vi "TimeLmtDialog.vi"(9 "time(s)":i32=5, 10 "Infoin":string="在这里填写显示的信息内容", 11 "title":string="提示信息") -> ()   [LabVIEW 2011]
panel:
  in  "ok":bool
  out "info":string
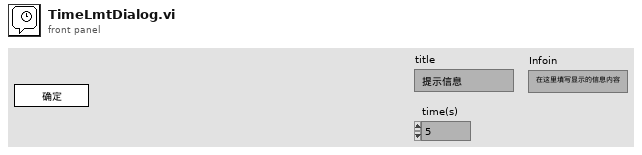
[diagram p1: front panel]
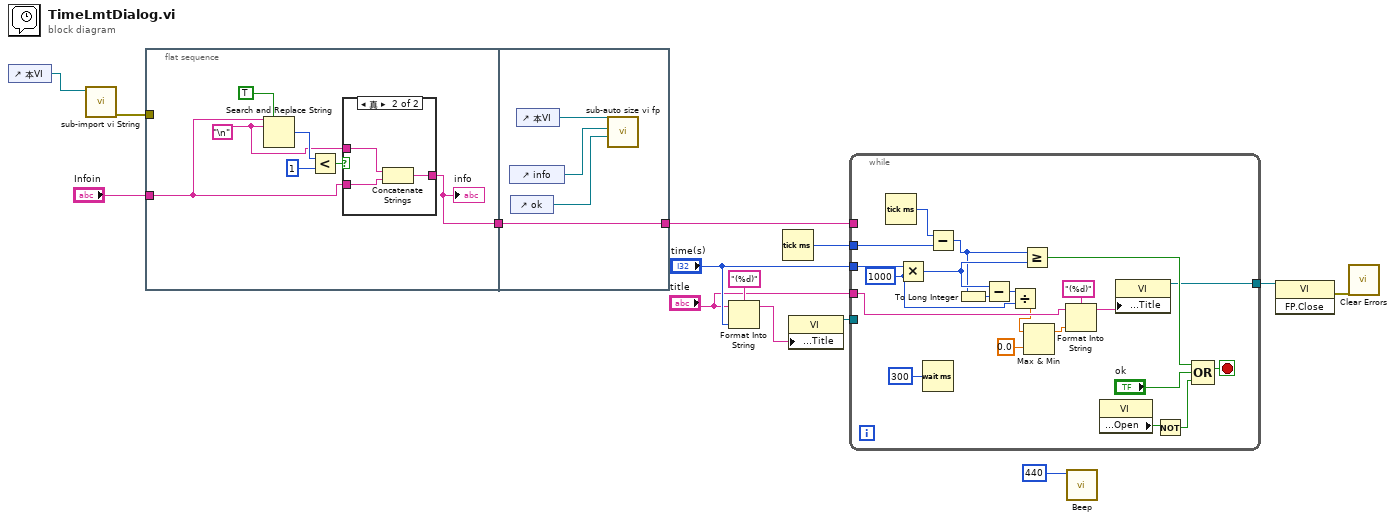
[diagram p0: block diagram]
diagram:
  n1 = control-ref of="本VI"() -> (w3:refnum<vi>)
  n2 = call "sub-import vi String.vi"("vi ref"=w3) -> ("error out"=w1:errorcluster)  [unwired: 10 in]
  n3 = flat-sequence {
    tunnel: "Infoin" -> [w15]
    tunnel: [w16] -> w2
    tunnel: w1 -> [_]
    tunnel: [w29] -> w5
    tunnel: w2 -> [w29]
    frame #0 {
      w17 = "\n"
      n4 = Search and Replace String(replace all?=TRUE ("替换全部？(F)"), input string=w15, search string=w17) -> (number of replacements=w20:i32)  [unwired: 5 in, 3 out]
      n5 = Less?(x=w20, y=1) -> (x < y?=w18:bool)
      n6 = case shown="真" w18 {
        tunnel: w15 -> [w22 w25]
        tunnel: w17 -> [_ w24]
        tunnel: [w22 w23] -> w16
        frame False {
        }
        frame True {
          n7 = Concatenate Strings(w24, w25) -> (w23:string)
        }
      }
      "info" <- w16
    }
    frame #1 {
      n8 = control-ref of="info"() -> (w26:refnum<vi>)
      n9 = control-ref of="ok"() -> (w27:refnum<vi>)
      n10 = control-ref of="本VI"() -> (w28:refnum<vi>)
      n11 = call "sub-auto size vi fp.vi"("btn ref"=w27, "str ref"=w26, "vi ref"=w28) -> ()  [unwired: 8 in, 1 out]
    }
  }
  n12 = Format Into String(format string="(%d)" ("格式字符串"), initial string="title", "time(s)") -> (resulting string=w11:string)  [unwired: 1 in, 1 out]
  n13 = Tick Count (ms)() -> (millisecond timer value=w9:u32)
  n14 = property class="VI"("Front Panel.Title"=w11) -> (reference out=w14:refnum<vi>)  [unwired: 2 in, 1 out]
  n15 = while {
    tunnel: w5 -> [_]
    tunnel: "time(s)" -> [w47]
    tunnel: w14 -> [_]
    tunnel: "title" -> [w39]
    tunnel: w9 -> [w48]
    tunnel: [w32] -> w8
    stop <- w44 stop-if-true
    w40 = 1000 ("y")
    n16 = Tick Count (ms)() -> (millisecond timer value=w49:u32)
    n17 = Multiply(x=w47, y=w40) -> (x*y=w43:i32)
    n18 = Wait (ms)(milliseconds to wait=u32 300 ("等待时间（毫秒）")) -> ()  [unwired: 1 out]
    n19 = Subtract(x=w49, y=w48) -> (x-y=w42:u32)
    n20 = To Long Integer(number=w42) -> (32bit integer=w33:i32)
    n21 = Subtract(x=w43, y=w33) -> (x-y=w41:i32)
    n22 = Divide(x=w41, y=w40) -> (x/y=w36:dbl)
    n23 = Greater Or Equal?(x=w42, y=w43) -> (x >= y?=w45:bool)
    n24 = Max & Min(x=w36, y=0.0) -> (max(x,y)=w34:dbl)  [unwired: 1 out]
    n25 = Format Into String(format string="(%d)" ("格式字符串"), initial string=w39, w34) -> (resulting string=w37:string)  [unwired: 1 in, 1 out]
    n26 = property class="VI"() -> ("Front Panel.Open"=w31:bool)  [unwired: 2 in, 2 out]
    n27 = property class="VI"("Front Panel.Title"=w37) -> (reference out=w32:refnum<vi>)  [unwired: 2 in, 1 out]
    n28 = Not(x=w31) -> (.not. x?=w30:bool)
    n29 = Compound Arithmetic op=OR(w45, "ok", w30) -> (w44:bool)
  }
  n30 = call <vilib>:"Beep.vi"("frequency (Hz)"=u32 440) -> ()  [unwired: 11 in]
  n31 = invoke class="VI" method="FP.Close"(reference=w8) -> (error out=w7:errorcluster)  [unwired: 2 in, 2 out]
  n32 = call <vilib>:"Clear Errors.vi"("error in (no error)"=w7) -> ()  [unwired: 6 in, 1 out]
